vi "Typedef to Ch settings.vi"(11 "Reply Payload":T1 {"Settings"."EEG Channels"."16 EEG Channels"."Channel No" step=1}) -> (2 "Referenced Channels":u16, 3 "Enabled Channels":u16)   [LabVIEW 2016, in "Acquisition.lvlib"]
uses:
  Acquisition.lvlib
  Settings Editor/Update Application Settings (Reply Payload)--cluster.ctl
  Settings Editor/Settings--cluster.ctl
  CML Shared/Signal Type--enum.ctl
  CML Shared/Calibration Values--cluster.ctl
  CML Shared/EEG Channel Settings.ctl
  CML Shared/CML Shared.lvlib
  Settings Editor/Settings Editor.lvlib
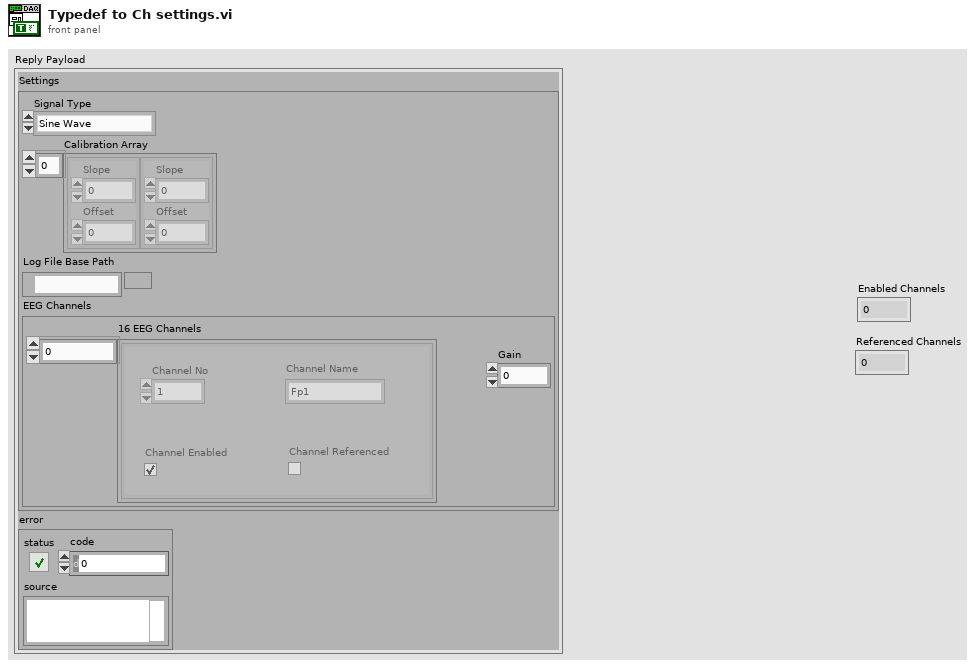
[diagram p1: front panel]
types:
  T1 = typedef "Settings Editor.lvlib/Update Application Settings (Reply Payload)--cluster.ctl" = cluster{"Settings":T2, "error":errorcluster}
  T2 = typedef "Settings Editor.lvlib/Settings--cluster.ctl" = cluster{"Signal Type":T3, "Calibration Array":T4[], "Log File Base Path":path, "EEG Channels":T5}
  T3 = typedef "CML Shared.lvlib/Signal Type--enum.ctl" = enum16{"Sine Wave", "Square with Noise"}
  T4 = typedef "CML Shared.lvlib/Calibration Values--cluster.ctl" = cluster{"Slope":dbl, "Offset":dbl}
  T5 = typedef "CML Shared.lvlib/EEG Channel Settings.ctl" = cluster{"16 EEG Channels":cluster{"Channel Name":string, "Channel No":u8, "Channel Enabled":bool, "Channel Referenced":bool}[], "Gain":u8}
  T6 = cluster{"Channel Name":string, "Channel No":u8, "Channel Enabled":bool, "Channel Referenced":bool}[]
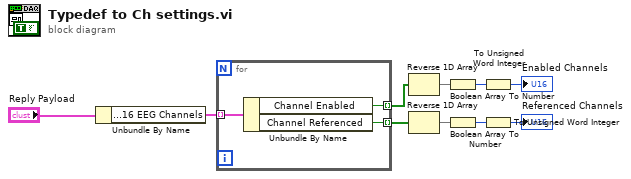
[diagram p0: block diagram]
diagram:
  n1 = Unbundle By Name("Reply Payload") -> ("Settings.EEG Channels.16 EEG Channels"=w7:T6)
  n2 = for {
    tunnel: w7 -> [w13] mode=indexing
    tunnel: [w12] -> w6 mode=indexing
    tunnel: [w11] -> w2 mode=indexing
    n3 = Unbundle By Name(w13) -> ("Channel Enabled"=w12:bool, "Channel Referenced"=w11:bool)
  }
  n4 = Reverse 1D Array(array=w6) -> (reversed array=w5:bool[])
  n5 = Reverse 1D Array(array=w2) -> (reversed array=w1:bool[])
  n6 = Boolean Array To Number(Boolean array=w5) -> (number=w8:u32)
  n7 = Boolean Array To Number(Boolean array=w1) -> (number=w4:u32)
  n8 = To Unsigned Word Integer(number=w8) -> (unsigned 16bit integer=→"Enabled Channels":u16)
  n9 = To Unsigned Word Integer(number=w4) -> (unsigned 16bit integer=→"Referenced Channels":u16)
